vi "Calculate Derived Stroker Digital Variables.vi"(8 "error in (no error)":errorcluster, 9 "Analog for digital calc":T9, 10 "Controller STAT2":T3 {"Tension Sub 2"."sys register" format="%04x"; "Tension Sub 1"."sys register" format="%04x"; "PSU"."sys register" format="%04x"; "solonoid"."valve status" format="%02x"; "solonoid"."sys register" format="%04x"; "pressure 2"."sys register" format="%04x"; "pressure 1"."sys register" format="%04x"; "Controller local"."High G monitoring" format="%02x"; "Controller local"."NA" format="%02x"; "Controller local"."GPIO values" format="%02x"; "Controller local"."Relay status" format="%02x"; "Controller local"."sys register" format="%04x"}, 11 "Selected Tool":T1) -> (0 "error out":errorcluster, 2 "Digital Variables Out":T2[](array[typedef]))   [LabVIEW 2011]
uses:
  Analog values for digital calculations.ctl
  Stroker/Stat def/Stroker system stat2.ctl
  LEINmaster/Nodes/Controller local stat2.ctl
  LEINmaster/Nodes/pressure stat2.ctl
  LEINmaster/Nodes/solonoid stat2.ctl
  LEINmaster/Nodes/PSU stat2.ctl
  LEINmaster/Nodes/tensionsub stat2.ctl
  Measurments Handling/Status Digitalish.ctl
  List of tools.ctl
  Variable List Tool Analog.ctl
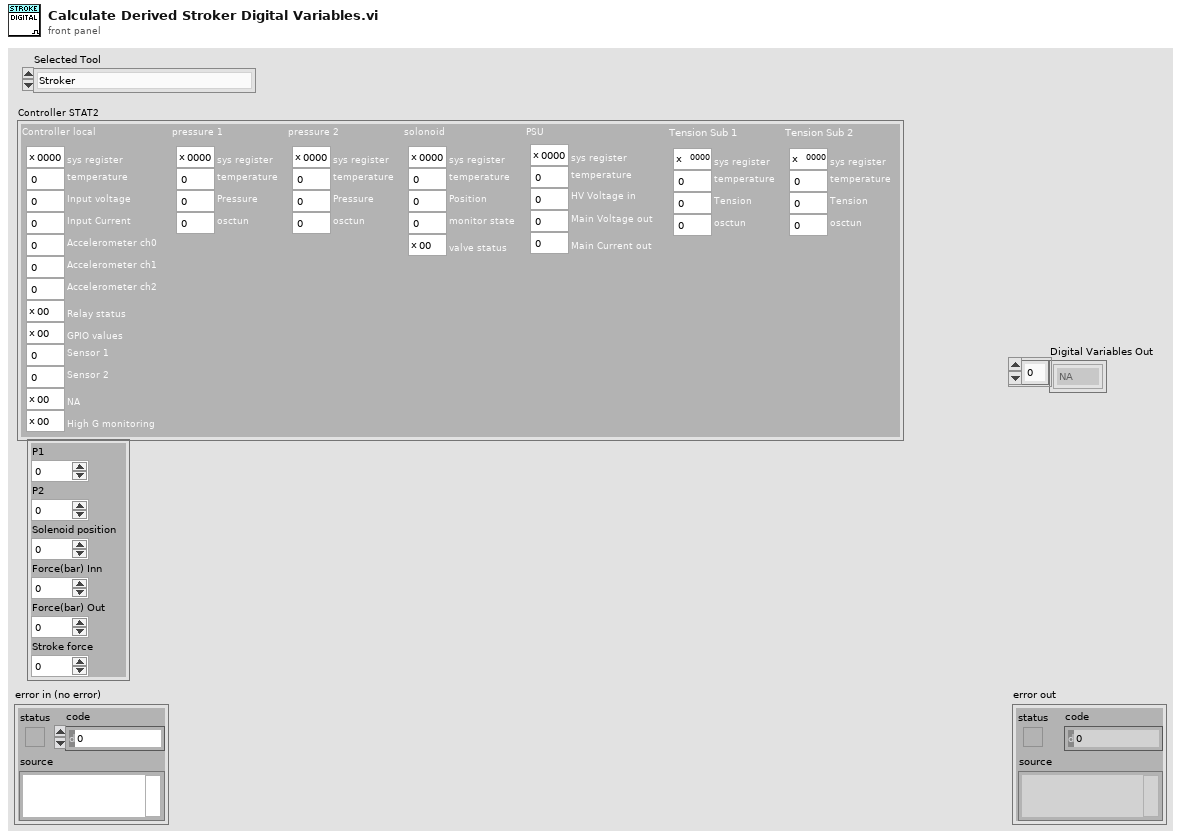
[diagram p1: front panel]
types:
  T1 = typedef "List of tools.ctl" = enum16{"Stroker", "Driller", "Tractor"}
  T2 = typedef "Status Digitalish.ctl" = enum16{"NA", "False", "True"}
  T3 = typedef "Stroker system stat2.ctl" = cluster{"Controller local":T4, "pressure 1":T5, "pressure 2":T5, "solonoid":T6, "PSU":T7, "Tension Sub 1":T8, "Tension Sub 2":T8}
  T4 = typedef "Controller local stat2.ctl" = cluster{"sys register":u16, "temperature":u16, "Input voltage":u16, "Input Current":u16, "Accelerometer ch0":u16, "Accelerometer ch1":u16, "Accelerometer ch2":u16, "Relay status":u8, "GPIO values":u8, "Sensor 1":i32, "Sensor 2":i32, "NA":u8, "High G monitoring":u8}
  T5 = typedef "pressure stat2.ctl" = cluster{"sys register":u16, "temperature":u16, "Pressure":u16, "osctun":u8}
  T6 = typedef "solonoid stat2.ctl" = cluster{"sys register":u16, "temperature":u16, "Position":i16, "monitor state":u8, "valve status":u8}
  T7 = typedef "PSU stat2.ctl" = cluster{"sys register":u16, "temperature":u16, "HV Voltage in":u16, "Main Voltage out":u16, "Main Current out":u16}
  T8 = typedef "tensionsub stat2.ctl" = cluster{"sys register":u16, "temperature":u16, "Tension":i16, "osctun":u8}
  T9 = typedef "Analog values for digital calculations.ctl" = cluster{"P1":dbl, "P2":dbl, "Solenoid position":dbl, "Force(bar) Inn":dbl, "Force(bar) Out":dbl, "Stroke force":dbl}
  T10 = typedef "Variable List Tool Analog.ctl" = enum16{"Tool Max Temperature", "Tool (Controller) Temperature", "Tool Supply Voltage", "Tool (Controller) Current", "Tool Acceleration X", "Tool Acceleration Y", "Tool Acceleration Z", "Tool Acceleration Sum", "Tool Inclination", "Tool Rotation", "Tool GP Sensor 1", "Tool GP Sensor 2", "Tool (Pressure 1) Temperature", "Tool Pressure 1 RAW", "Tool (Pressure 2) Temperature", "Tool Pressure 2 RAW", "Tool (Solenoid) Temperature", "Tool Solenoid Position", "PSU Temp", "Head Voltage", "PSU Main Voltage out", "PSU Main Current out", "Upper Tension Sub Temp", "Tool Upper Tension Sub Raw", "Lower Tension Sub Temp", "Tool Lower Tension Sub Raw", "Tool Var27 - Reserved", "Tool Var28 - Reserved", "Tool Var29 - Reserved", "Tool Var30 - Reserved", "Stroke Extension", "Stroke In Force", "Stroke Out Force", "Stroke Force", "Stroker Pressure 1", "Stroker Pressure 2", "Stroker Upper Tension Sub", "Stroker Lower Tension Sub", "Stroker Var09 - Reserved", "Stroker Var10 - Reserved", "Tractor Upper Tension Sub", "Tractor Lower Tension Sub", "Tractor Var03 - Reserved", "Tractor Var04 - Reserved", "Tool Temperature sensor", "Tool Motor Voltage", "Tool Motor Current", "Tool Motor Torque", "Tool weight on bit", "Tool Motor RPM"}
  T11 = typedef "Stat2 system task info.ctl" = cluster{"Task":bool, "Task error":bool, "Task cnt.":u8, "Job 0":bool, "User":bool}
  T12 = typedef "Options  All pages and custom.ctl" = cluster{"P 1 (App)":T13, "P 2":T14, "P 3":T15, "P 4":T18, "P 5":T23, "P 6 (Err)":T24, "P 7 (Expert)":T25, "P 8 (Depth)":T27, "C 1":T28, "C 2":T29}
  T13 = typedef "Options Page 1 (App).ctl" = cluster{"Result files":path, "PCP Interface":string, "Tractor/Stroker Interface":string, "Tractor Interface":string, "Modem Status Interface":string, "Audible Alarm":bool, "Force alarm on Technical":bool, "Force alarm on HH":bool, "Force alarm on LL":bool, "Force alarm on H":bool, "Force alarm on L":bool}
  T14 = typedef "Options Page 2.ctl" = cluster{"Solenoid & Relay latching time":u16, "Tractor relay 1":dbl, "Tractor relay 2":dbl, "Tractor Solenoid limit":dbl}
  T15 = typedef "Options Page 3.ctl" = cluster{"Min resistance":dbl, "Max resistance":dbl, "Head voltage range":T16, "Max voltage jump":dbl, "Maximum resistance change":dbl, "Start Telemetry Voltage":dbl, "Start Telemetry Timeout":dbl, "Start Motor Voltage":dbl, "Stop Motor Voltage":dbl, "Pass Mode Warning Voltage":dbl, "Relay Switch Voltage":dbl, "Relay Status Loss Voltage":dbl, "Samples to average":i32, "PSU type DO NOT USE":T17, "Magna OVP":dbl, "Magna Current Limit":dbl}
  T16 = typedef "PCP type List.ctl" = enum16{"0 - 350V", "0 - 450V", "0 - 600V"}
  T17 = typedef "PSU Type.ctl" = enum16{"Unipower", "Magna 8.3A", "Magna 12A", "None"}
  T18 = typedef "Options Page 4.ctl" = cluster{"Solenoid & Relay latching time":u16, "Stroker relay 1":dbl, "Stroker Relay 2":dbl, "Stroker Solenoid limit":dbl, "Force det.":T19, "Stroke force lim.":dbl, "Anchor Enabled Pressure":dbl, "Tacometer puls":dbl, "Default anchor behavior":T20, "Default stroker behavior":T21, "Default stroker force limit (tonne)":dbl, "Slips Size":T22}
  T19 = typedef "Stroke force selector.ctl" = enum16{"Stroke in = node 1", "Strok out = node 1"}
  T20 = typedef "Default anchor behavior.ctl" = enum16{"Do nothing", "Set Anchor", "Release Anchor"}
  T21 = typedef "Default stroker behavior.ctl" = enum16{"Do nothing", "Stop", "Go Out", "Go In"}
  T22 = typedef "Slips Type Radio.ctl" = enum32{"No Selection", "338 MRS", "3,9 MRS"}
  T23 = typedef "Options Page 5.ctl" = cluster{"Solenoid & Relay latching time":u16, "Driller relay 1":dbl, "Driller Relay 2":dbl, "Driller  Solenoid limit":dbl}
  T24 = typedef "Options Page 6 (Err).ctl" = cluster{"Error and event files":path}
  T25 = typedef "Options Page 7 (Expert).ctl" = cluster{"Show Debug":bool, "Log debug messages":bool, "Additional debug messages":bool, "Start Beagle with Simulator data":bool, "Workshop mode":bool, "Modem baud":u16, "enumCANCOM":bool, "Modem sim":T26, "Telemetry Timeout Disable":i32, "Buffer size":i32, "Upd regular data":bool, "Cable comp":cluster{"VMOD1 Voltage(V)":dbl, "VMOD2 Voltage(V)":dbl}}
  T26 = typedef "Modem simulation setup.ctl" = cluster{"Modem dealay sim":bool, "Sim baud Tx":u16, "Bit Error fraction Tx":dbl, "Sim baud Rx":u16, "Bit Error fraction Rx":dbl}
  T27 = typedef "Options Page 8 (Depth).ctl" = cluster{"Winch Spool Circumference":dbl, "Winch Pulses per Revolution":dbl, "Current Depth":dbl}
  T28 = typedef "Options Custom 1.ctl" = cluster{"Depth Updated":bool, "Depth Offset":dbl}
  T29 = typedef "Options Custom 2.ctl" = cluster{"Placeholder":bool}
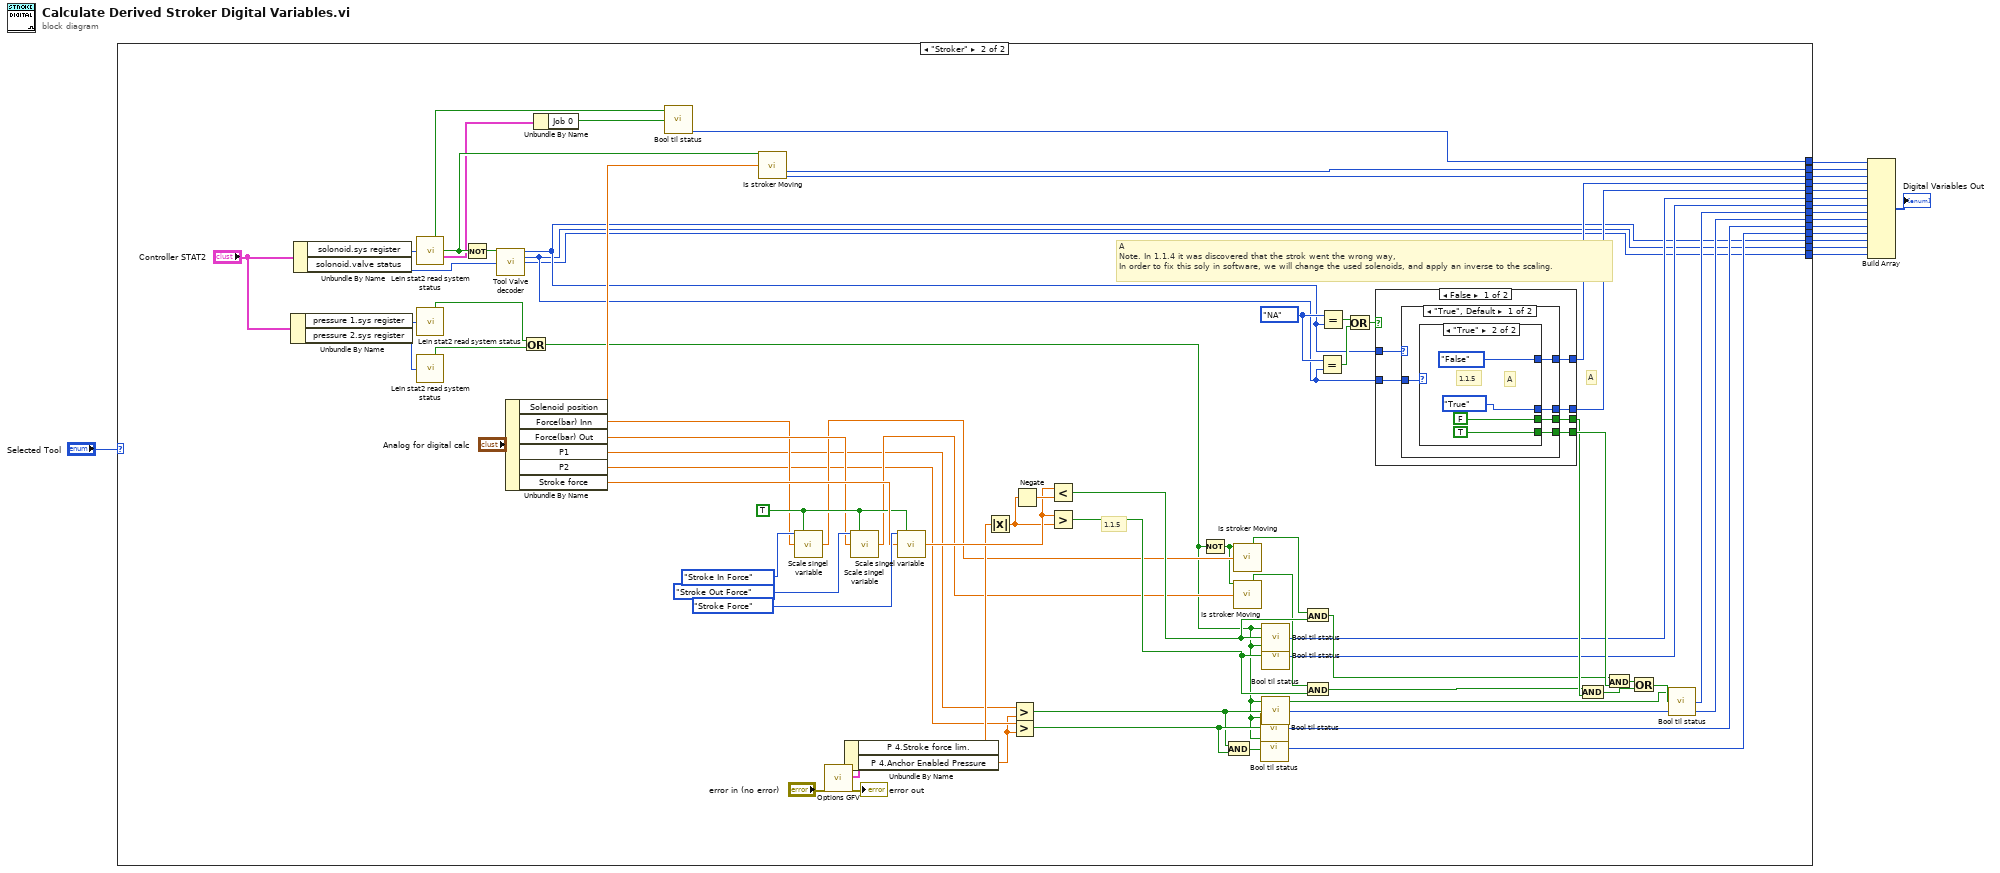
[diagram p0: block diagram]
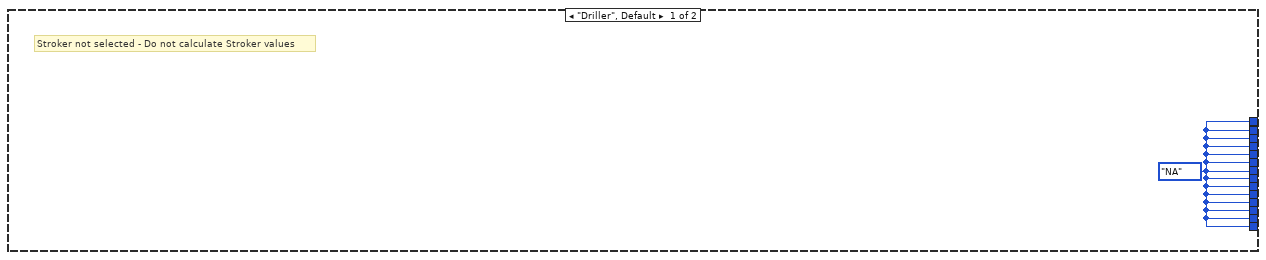
[diagram p2: hidden frame]
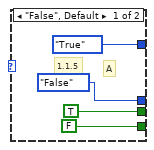
[diagram p3: hidden frame]
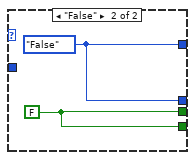
[diagram p4: hidden frame]
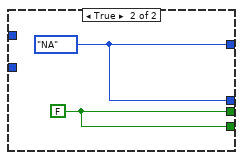
[diagram p5: hidden frame]
diagram:
  n1 = case shown="\"Stroker\"" "Selected Tool" {
    tunnel: [w17 w84] -> w16
    tunnel: [w17 w83] -> w15
    tunnel: [w17 w44] -> w14
    tunnel: [w17 w43] -> w13
    tunnel: [w17 w41] -> w12
    tunnel: [w17 w40] -> w11
    tunnel: [w17 w39] -> w10
    tunnel: [w17 w38] -> w9
    tunnel: [w17 w37] -> w8
    tunnel: [w17 w36] -> w7
    tunnel: [w17 w21] -> w4
    tunnel: [w17 w20] -> w3
    tunnel: [w17 w19] -> w2
    tunnel: [w17 w18] -> w1
    frame "Driller", Default {
      w17 = Status_Digitalish."NA" ("Increase")
      # "Stroker not selected - Do not calculate Stroker values"
    }
    frame "Stroker" {
      w72 = TRUE ("Tool")
      w45 = Status_Digitalish."NA" ("x")
      # "A\nNote. In 1.1.4 it was discovered that the strok went the wrong way,\nIn order to fix this soly in software, we will change the used solenoids, and apply an inverse to the scaling."
      # "1.1.5"
      # "A"
      n2 = Unbundle By Name("Controller STAT2") -> ("pressure 1.sys register"=w30:u16, "pressure 2.sys register"=w31:u16)
      n3 = Unbundle By Name("Controller STAT2") -> ("solonoid.sys register"=w26:u16, "solonoid.valve status"=w29:u8)
      n4 = call "Lein stat2 read system status.vi"("sys register"=w26) -> ("Force NA"=w22:bool, "Connected"=w25:bool, "Task"=w24:T11)  [unwired: 7 in, 5 out]
      n5 = call "Lein stat2 read system status.vi"("sys register"=w30) -> ("Force NA"=w33:bool)  [unwired: 7 in, 7 out]
      n6 = call "Lein stat2 read system status.vi"("sys register"=w31) -> ("Force NA"=w32:bool)  [unwired: 7 in, 7 out]
      n7 = Not(x=w25) -> (.not. x?=w34:bool)
      n8 = call "Tool Valve decoder.vi"("Force NA(F)"=w34, "Valve Relay code"=w29) -> ("Valve LSB(0)"=w20:T2, "Valve 1"=w19:T2, "Valve 2"=w18:T2)  [unwired: 9 in, 2 out]
      n9 = Unbundle By Name("Analog for digital calc") -> ("Solenoid position"=w35:dbl, "Force(bar) Inn"=w68:dbl, "Force(bar) Out"=w70:dbl, "P1"=w53:dbl, "P2"=w54:dbl, "Stroke force"=w73:dbl)
      n10 = Or(x=w33, y=w32) -> (x .or. y?=w28:bool)
      n11 = Unbundle By Name(w24) -> ("Job 0"=w23:bool)
      n12 = call "Bool til status.vi"("Force NA(F)"=w22, "Boolean"=w23) -> ("Status"=w21:T2)  [unwired: 7 in]
      n13 = call "Is stroker Moving.vi"("Connected"=w25, "Position"=w35) -> ("Increase"=w84:T2, "Decrease"=w83:T2)  [unwired: 8 in, 4 out]
      n14 = call "Scale singel variable.vi"("Index"=Variable_List_Tool_Analog."Stroke In Force" ("Variable ID"), "Tool"=w72, "Val in"=w68) -> ("Val out"=w69:dbl)  [unwired: 11 in, 1 out]
      n15 = call "Options GFV.vi"("error in (no error)"="error in (no error)") -> ("Options"=w50:T12, "error out"=→"error out":errorcluster)  [unwired: 16 in, 1 out]
      n16 = Unbundle By Name(w50) -> ("P 4.Stroke force lim."=w74:dbl, "P 4.Anchor Enabled Pressure"=w52:dbl)
      n17 = call "Scale singel variable.vi"("Index"=Variable_List_Tool_Analog."Stroke Out Force" ("Variable ID"), "Tool"=w72, "Val in"=w70) -> ("Val out"=w71:dbl)  [unwired: 11 in, 1 out]
      n18 = call "Scale singel variable.vi"("Index"=Variable_List_Tool_Analog."Stroke Force" ("Variable ID"), "Tool"=w72, "Val in"=w73) -> ("Val out"=w76:dbl)  [unwired: 11 in, 1 out]
      n19 = Absolute Value(x=w74) -> (abs(x)=w75:dbl)
      n20 = Greater?(x=w53, y=w52) -> (0:w55:bool)
      n21 = Greater?(x=w54, y=w52) -> (0:w56:bool)
      n22 = Negate(x=w75) -> (-x=w77:dbl)
      n23 = Less?(x=w76, y=w77) -> (x < y?=w79:bool)
      n24 = Greater?(x=w76, y=w75) -> (0:w78:bool)
      n25 = Not(x=w28) -> (.not. x?=w59:bool)
      n26 = And(x=w55, y=w56) -> (x .and. y?=w57:bool)
      n27 = call "Is stroker Moving.vi"("Connected"=w59, "Position"=w69) -> ("Decrease"=w58:bool)  [unwired: 8 in, 5 out]
      n28 = call "Is stroker Moving.vi"("Connected"=w59, "Position"=w71) -> ("Decrease"=w60:bool)  [unwired: 8 in, 5 out]
      n29 = call "Bool til status.vi"("Force NA(F)"=w28, "Boolean"=w56) -> ("Status"=w37:T2)  [unwired: 7 in]
      n30 = call "Bool til status.vi"("Force NA(F)"=w28, "Boolean"=w57) -> ("Status"=w36:T2)  [unwired: 7 in]
      n31 = call "Bool til status.vi"("Force NA(F)"=w28, "Boolean"=w79) -> ("Status"=w41:T2)  [unwired: 7 in]
      n32 = call "Bool til status.vi"("Force NA(F)"=w28, "Boolean"=w78) -> ("Status"=w40:T2)  [unwired: 7 in]
      n33 = call "Bool til status.vi"("Force NA(F)"=w28, "Boolean"=w55) -> ("Status"=w38:T2)  [unwired: 7 in]
      n34 = And(x=w58, y=w79) -> (x .and. y?=w62:bool)
      n35 = And(x=w60, y=w78) -> (x .and. y?=w61:bool)
      n36 = Equal?(x=w45, y=w19) -> (x = y?=w48:bool)
      n37 = Equal?(x=w45, y=w20) -> (x = y?=w47:bool)
      n38 = Or(x=w47, y=w48) -> (x .or. y?=w46:bool)
      n39 = case shown="False" w46 {
        tunnel: w20 -> [w90 _]
        tunnel: [w89 w107] -> w44
        tunnel: [w88 w107] -> w43
        tunnel: w19 -> [w87 _]
        tunnel: [w86 w106] -> w65
        tunnel: [w85 w106] -> w67
        frame False {
          n40 = case shown="\"True\", Default" w90 {
            tunnel: [w95 w105] -> w89
            tunnel: [w94 w105] -> w88
            tunnel: w87 -> [w93 _]
            tunnel: [w92 w104] -> w86
            tunnel: [w91 w104] -> w85
            frame "True", Default {
              n41 = case shown="\"True\"" w93 {
                tunnel: [Status_Digitalish."True" ("Valve LSB(0)") Status_Digitalish."False" ("Valve LSB(0)")] -> w95
                tunnel: [Status_Digitalish."False" ("Valve LSB(0)") Status_Digitalish."True" ("Valve LSB(0)")] -> w94
                tunnel: [TRUE FALSE] -> w92
                tunnel: [FALSE TRUE] -> w91
                frame "False", Default {
                  # "A"
                  # "1.1.5"
                }
                frame "True" {
                  # "A"
                  # "1.1.5"
                }
              }
            }
            frame "False" {
              w104 = FALSE
              w105 = Status_Digitalish."False" ("Valve LSB(0)")
            }
          }
        }
        frame True {
          w106 = FALSE
          w107 = Status_Digitalish."NA" ("Valve LSB(0)")
        }
      }
      n42 = And(x=w61, y=w65) -> (x .and. y?=w64:bool)
      n43 = And(x=w62, y=w67) -> (x .and. y?=w66:bool)
      n44 = Or(x=w66, y=w64) -> (x .or. y?=w63:bool)
      n45 = call "Bool til status.vi"("Force NA(F)"=w28, "Boolean"=w63) -> ("Status"=w39:T2)  [unwired: 7 in]
    }
  }
  n46 = Build Array(w4, w16, w15, w14, w13, w12, w11, w10, w9, w8, w7, w3, w2, w1) -> (→"Digital Variables Out":T2[])
